vi "Check if Sequence Should Execute.vi"(10 "Current time":timestamp, 11 "Settings in":T1) -> (1 "Use Default Values":bool, 2 "Execute Sequence":bool, 3 "Settings out":T1)   [LabVIEW 2020, in "Sequencer with Output Values.lvlib" / "Sequencer with Output Values.lvclass"]
uses:
  Sequencer with Output Values.lvclass
  Params.ctl
  Step Settings.ctl
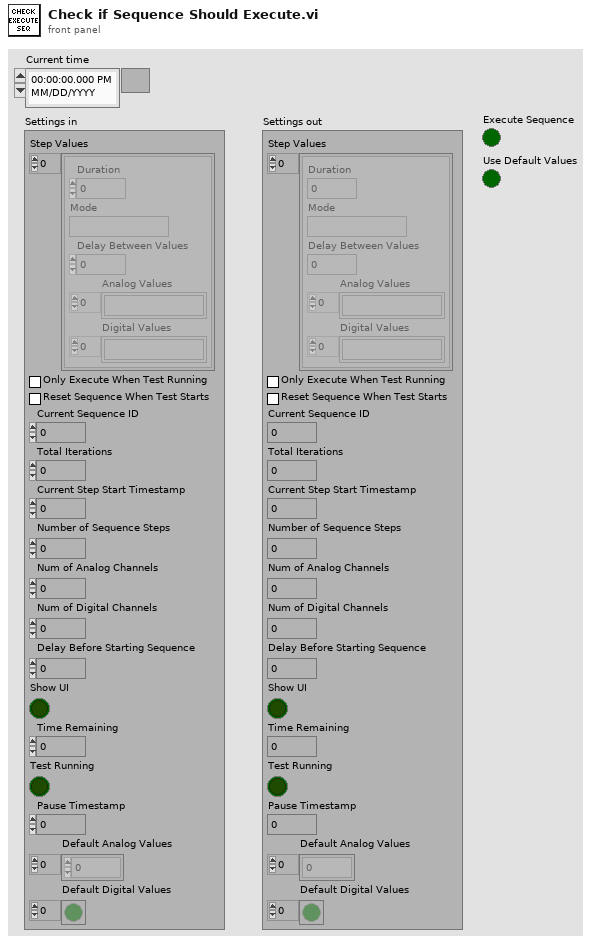
[diagram p1: front panel]
types:
  T1 = typedef "Sequencer with Output Values.lvlib/Sequencer with Output Values.lvclass/Params.ctl" = cluster{"Step Values":T2[], "Only Execute When Test Running":bool, "Reset Sequence When Test Starts":bool, "Current Sequence ID":u32, "Total Iterations":u32, "Current Step Start Timestamp":dbl, "Number of Sequence Steps":i32, "Num of Analog Channels":i32, "Num of Digital Channels":i32, "Delay Before Starting Sequence":dbl, "Show UI":bool, "Time Remaining":dbl, "Test Running":bool, "Pause Timestamp":dbl, "Default Analog Values":dbl[], "Default Digital Values":bool[]}
  T2 = typedef "Sequencer with Output Values.lvlib/Sequencer with Output Values.lvclass/Step Settings.ctl" = cluster{"Duration":dbl, "Mode":string, "Delay Between Values":dbl, "Analog Values":string[], "Digital Values":string[]}
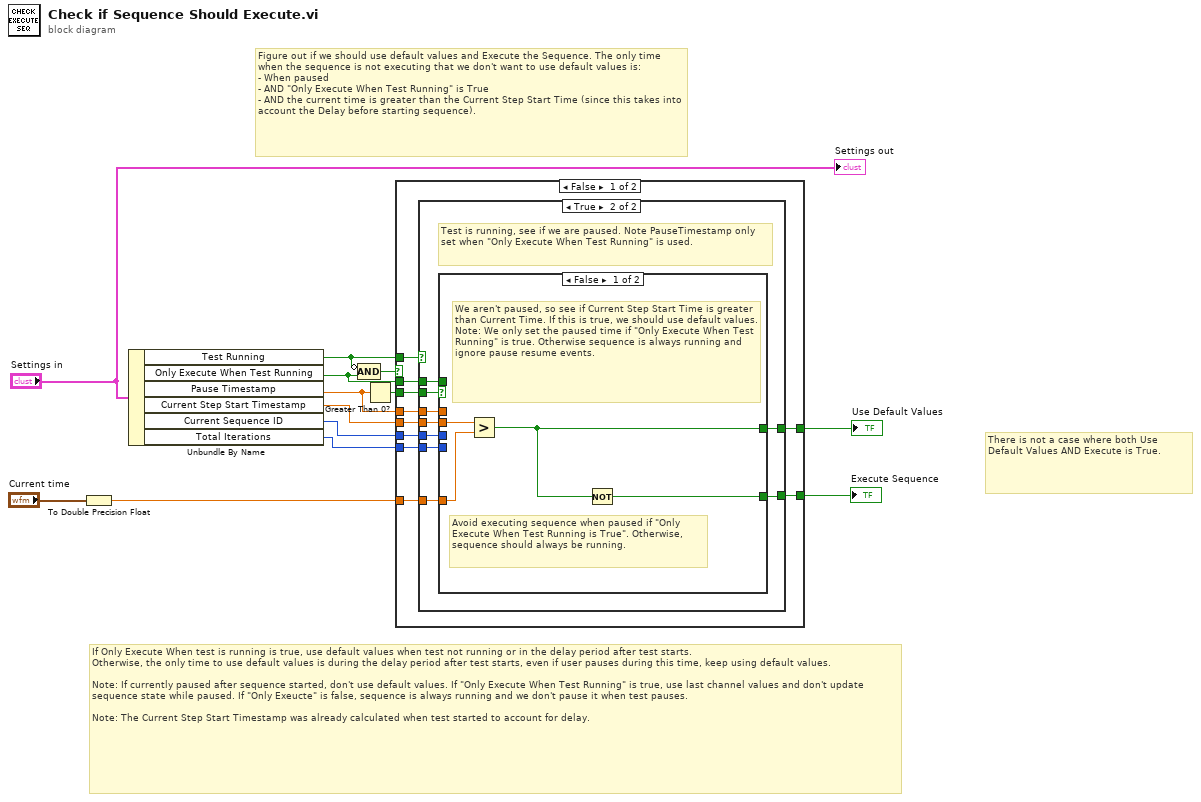
[diagram p0: block diagram]
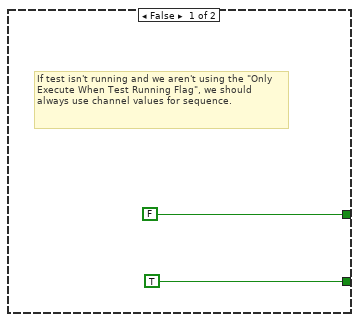
[diagram p2: hidden frame]
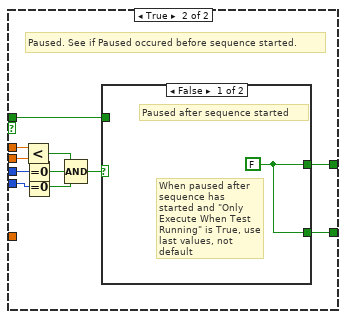
[diagram p3: hidden frame]
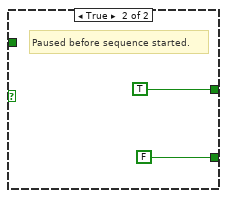
[diagram p4: hidden frame]
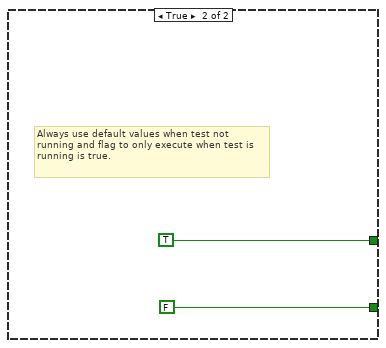
[diagram p5: hidden frame]
diagram:
  # "There is not a case where both Use Default Values AND Execute is True."
  # "Figure out if we should use default values and Execute the Sequence. The only time when the sequence is not executing that we don't want to use default values is:\n- When paused \n- AND \"Only Execute When Test Running\" is True \n- AND the current time is greater than the Current Step Start Time (since this takes into account the Delay before starting sequence)."
  # "If Only Execute When test is running is true, use default values when test not running or in the delay period after test starts.\nOtherwise, the only time to use default values is during the delay period after test starts, even if user pauses during this time, keep using default values.\n\nNote: If currently paused after sequence started, don't use default values. If \"Only Execute When Test Running\" is true, use last channel values and don't update sequence state while paused. If \"Only Exeucte\" is false, sequence is always running and we don't pause it when test pauses.\n\nNote: The Current Step Start Timestamp was already calculated when test started to account for delay."
  n1 = To Double Precision Float(number="Current time") -> (double precision float=w3:dbl)
  n2 = Unbundle By Name("Settings in") -> ("Test Running"=w7:bool, "Only Execute When Test Running"=w6:bool, "Pause Timestamp"=w5:dbl, "Current Step Start Timestamp"=w4:dbl, "Current Sequence ID"=w2:u32, "Total Iterations"=w1:u32)
  n3 = Compound Arithmetic op=AND(invert w7, w6) -> (w11:bool)
  n4 = Greater Than 0?(x=w5) -> (x > 0?=w12:bool)
  n5 = case shown="False" w11 {
    tunnel: w12 -> [w18 _]
    tunnel: w4 -> [w23 _]
    tunnel: w3 -> [w22 _]
    tunnel: [w20 TRUE] -> w8
    tunnel: w7 -> [w21 _]
    tunnel: [w19 FALSE] -> w9
    tunnel: w5 -> [w17 _]
    tunnel: w6 -> [w16 _]
    tunnel: w2 -> [w15 _]
    tunnel: w1 -> [w14 _]
    frame False {
      n6 = case shown="True" w21 {
        tunnel: w23 -> [_ w34]
        tunnel: w22 -> [_ w33]
        tunnel: [FALSE w31] -> w20
        tunnel: [TRUE w30] -> w19
        tunnel: w18 -> [_ w32]
        tunnel: w17 -> [_ w29]
        tunnel: w16 -> [_ w28]
        tunnel: w15 -> [_ w27]
        tunnel: w14 -> [_ w26]
        frame False {
          # "If test isn't running and we aren't using the \"Only Execute When Test Running Flag\", we should always use channel values for sequence."
        }
        frame True {
          # "Test is running, see if we are paused. Note PauseTimestamp only set when \"Only Execute When Test Running\" is used."
          n7 = case shown="False" w32 {
            tunnel: w34 -> [w38 w48]
            tunnel: w33 -> [w37 _]
            tunnel: [w36 w47] -> w31
            tunnel: [w35 w46] -> w30
            tunnel: w29 -> [_ w49]
            tunnel: w28 -> [_ w45]
            tunnel: w27 -> [_ w43]
            tunnel: w26 -> [_ w41]
            frame False {
              # "Avoid executing sequence when paused if \"Only Execute When Test Running is True\". Otherwise, sequence should always be running."
              # "We aren't paused, so see if Current Step Start Time is greater than Current Time. If this is true, we should use default values. Note: We only set the paused time if \"Only Execute When Test Running\" is true. Otherwise sequence is always running and ignore pause resume events."
              n8 = Greater?(x=w38, y=w37) -> (0:w36:bool)
              n9 = Not(x=w36) -> (.not. x?=w35:bool)
            }
            frame True {
              # "Paused. See if Paused occured before sequence started."
              n10 = Less?(x=w49, y=w48) -> (x < y?=w44:bool)
              n11 = Equal To 0?(x=w43) -> (x = 0?=w42:bool)
              n12 = Equal To 0?(x=w41) -> (x = 0?=w40:bool)
              n13 = Compound Arithmetic op=AND(w44, w42, w40) -> (w39:bool)
              n14 = case shown="False" w39 {
                tunnel: [w50 TRUE] -> w47
                tunnel: [w50 FALSE] -> w46
                tunnel: w45 -> [_ _]
                frame False {
                  w50 = FALSE
                  # "When paused after sequence has started and \"Only Execute When Test Running\" is True, use last values, not default"
                  # "Paused after sequence started"
                }
                frame True {
                  # "Paused before sequence started."
                }
              }
            }
          }
        }
      }
    }
    frame True {
      # "Always use default values when test not running and flag to only execute when test is running is true."
    }
  }
  "Execute Sequence" <- w9
  "Use Default Values" <- w8
  "Settings out" <- "Settings in"
